vi "closed_loop_starter.vi"() -> ()   [LabVIEW 2018]
uses:
  Controls/StatisticsData.ctl
  Classes/WavefrontCorrector/WavefrontCorrector.lvclass
  Classes/CorrectionDataManager/CorrectionDataManager.lvclass
  Classes/Camera/Camera.lvclass
  Classes/WavefrontCorrectorSet/WavefrontCorrectorSet.lvclass
  Classes/Image/Image.lvclass
  Classes/ClosedLoopSmoothing/ClosedLoopSmoothing.lvclass
  Classes/HasoSlopes/HasoSlopes.lvclass
  Controls/SlopesPostProcessorList - Filter.ctl
  Controls/InteractionMatrixToCommandMatrixParameters.ctl
  Classes/Phase/Phase.lvclass
  Controls/WavefrontReconstructionMode.ctl
  Classes/Pupil/Pupil.lvclass
panel:
  in  "set_init_state_from_config_file":bool
  out "Phase values":sgl[][](graph)
  out "StatisticsData":T1
  out "Gain out":dbl min=0.0 max=1.0
  in  "Gain in":dbl min=0.0 max=1.0
  in  "Init":bool
  in  "Start Loop":bool
  in  "Exit":bool
  in  "Stop Loop":bool
  out "Camera image":u32[][](graph)
  in  "Interaction matrix file path":path
  out "error out":errorcluster
  out "ActuatorsNumber":i32
  in  "Wavefront configuration file path":path
  in  "Haso configuration file path":path
  # "This example is Hardware-dependant, \nplease use your own Haso and corrector configuration file and acquisition system, as well as your correction data backup file.\nIf you don't have a correction data backup file, please run the correction data example."
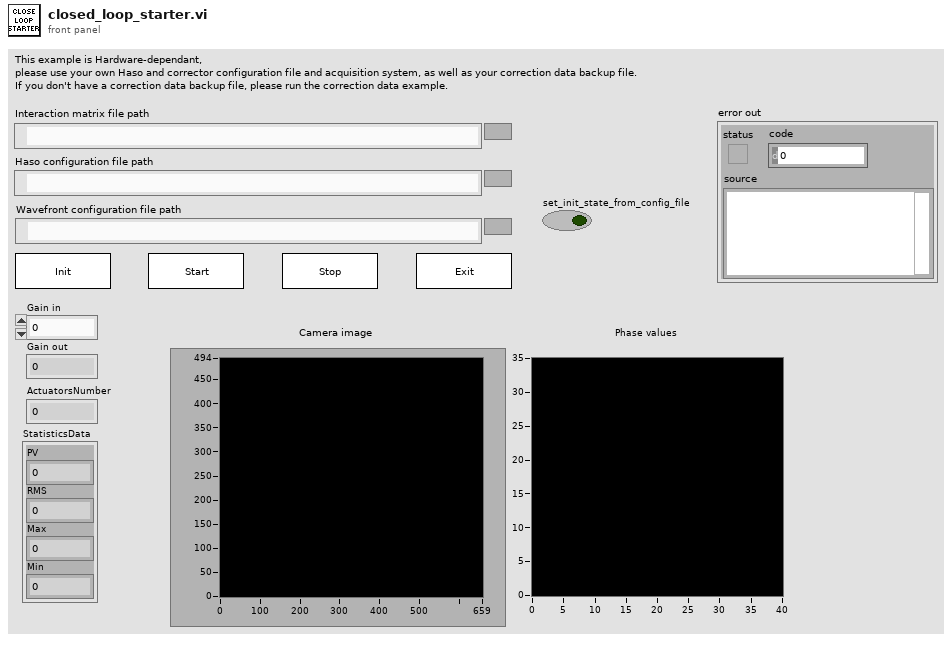
[diagram p1: front panel]
types:
  T1 = typedef "StatisticsData.ctl" = cluster{"PV":sgl, "RMS":dbl, "Max":sgl, "Min":sgl}
  T2 = typedef "SlopesPostProcessorList - Filter.ctl" = cluster{"tiltx":bool, "tilty":bool, "curv":bool, "astig0":bool, "astig45":bool, "others":bool}
  T3 = typedef "InteractionMatrixToCommandMatrixParameters.ctl" = cluster{"Number of kept modes":i32, "Tilt filtering":bool}
  T4 = typedef "WavefrontReconstructionMode.ctl" = enum16{"None", "Modal_Legendre", "Modal_Zernike", "Zonal", "Modal_Zonal_Zernike", "Modal_Zonal_Legendre"}
  T5 = typedef "HasoSpecifications.ctl" = cluster{"Serial number":string, "Revision":string, "Model":string, "Dimensions_um":T6, "Pixel position for alignment":T8, "Radius tolerance":u16, "Default start subaperture_sspp":T7, "Lower calibration wavelength_nm":dbl, "Upper calibration wavelength_nm":dbl, "Black subaperture position_sspp":T7, "TiltLimit_mrad":dbl, "Radius_m":dbl, "Smearing limit wavelength_nm":dbl, "Smearing limit exposure duration_us":dbl, "Focal_um":dbl}
  T6 = typedef "General dimensions definition.ctl" = cluster{"Size":T7, "Step":T8}
  T7 = typedef "Point2D.ctl" = cluster{"X":u32, "Y":u32}
  T8 = typedef "Point2Df.ctl" = cluster{"X":sgl, "Y":sgl}
  T9 = typedef "Data alignment enum.ctl" = enum16{"8", "16", "32"}
  T10 = typedef "Wavefront Corrector Position.ctl" = sgl[]
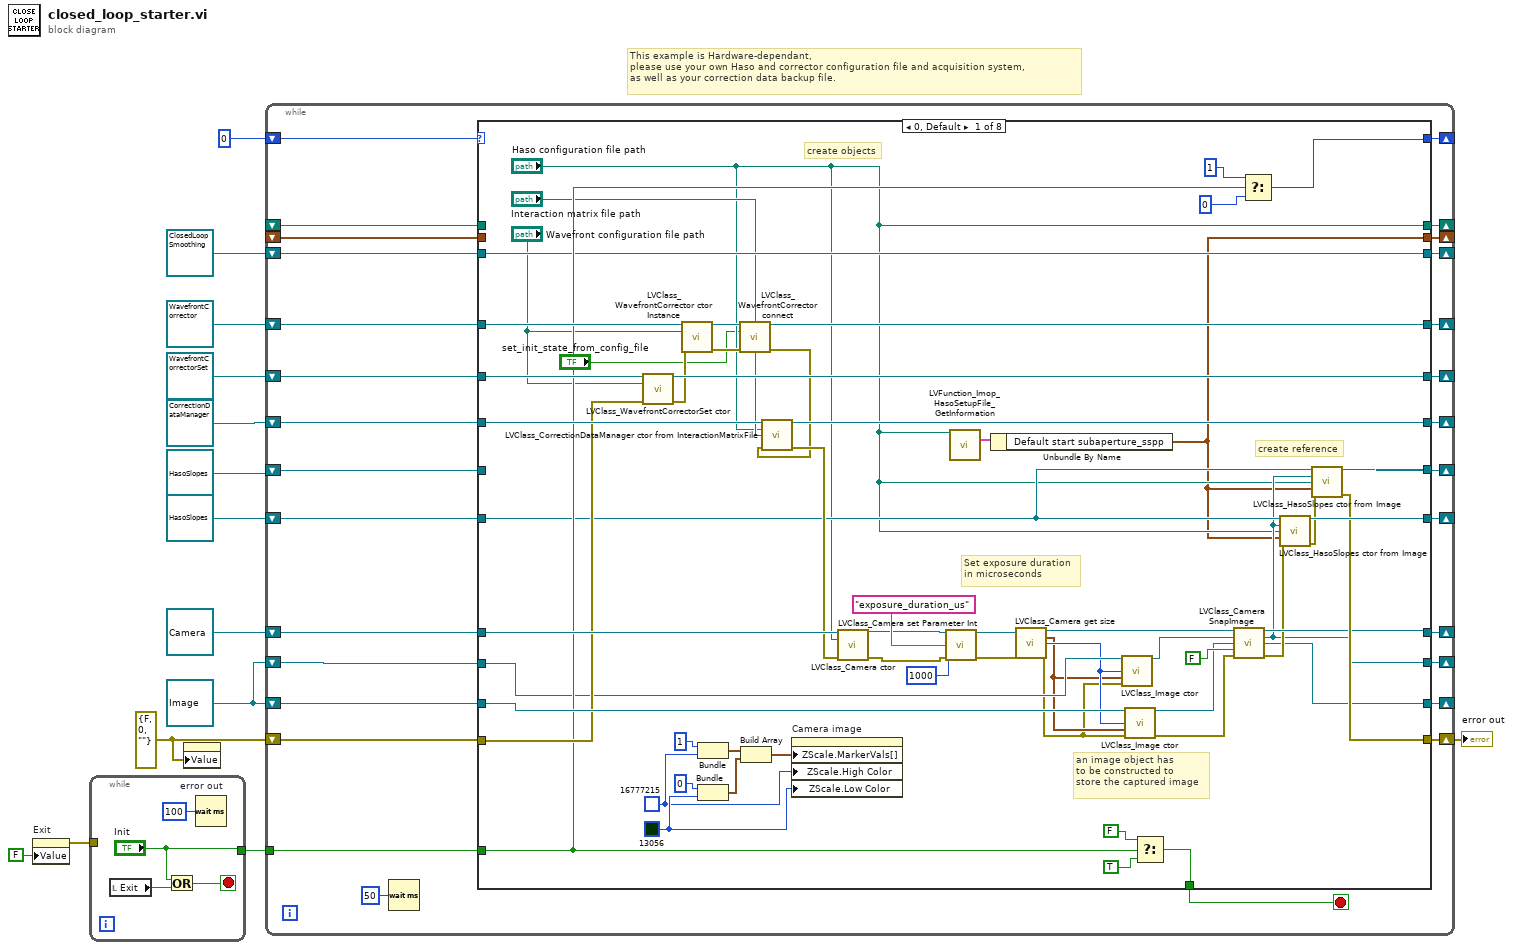
[diagram p0: block diagram]
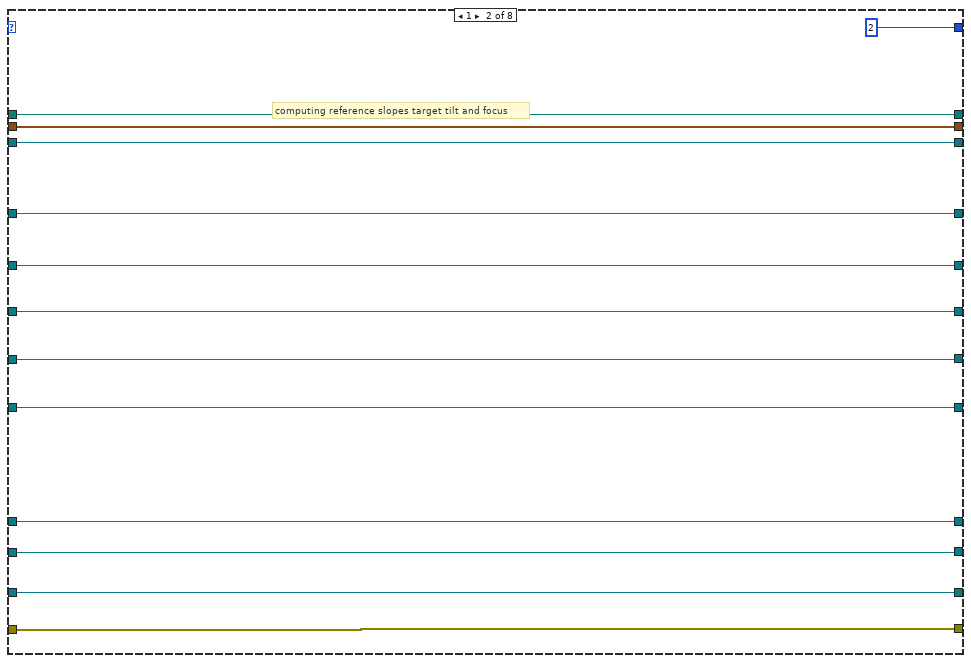
[diagram p2: hidden frame]
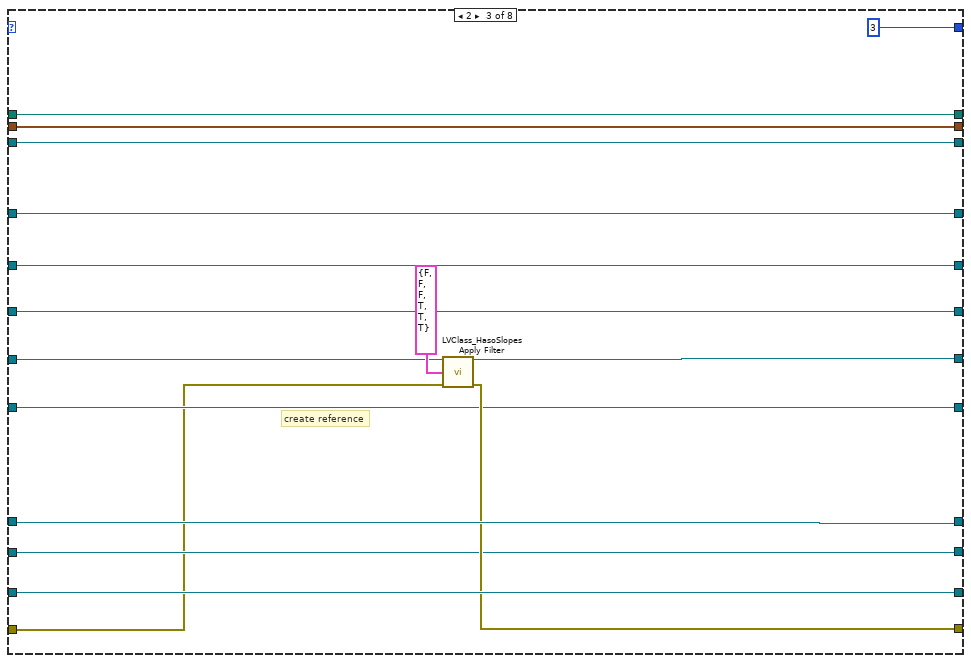
[diagram p3: hidden frame]
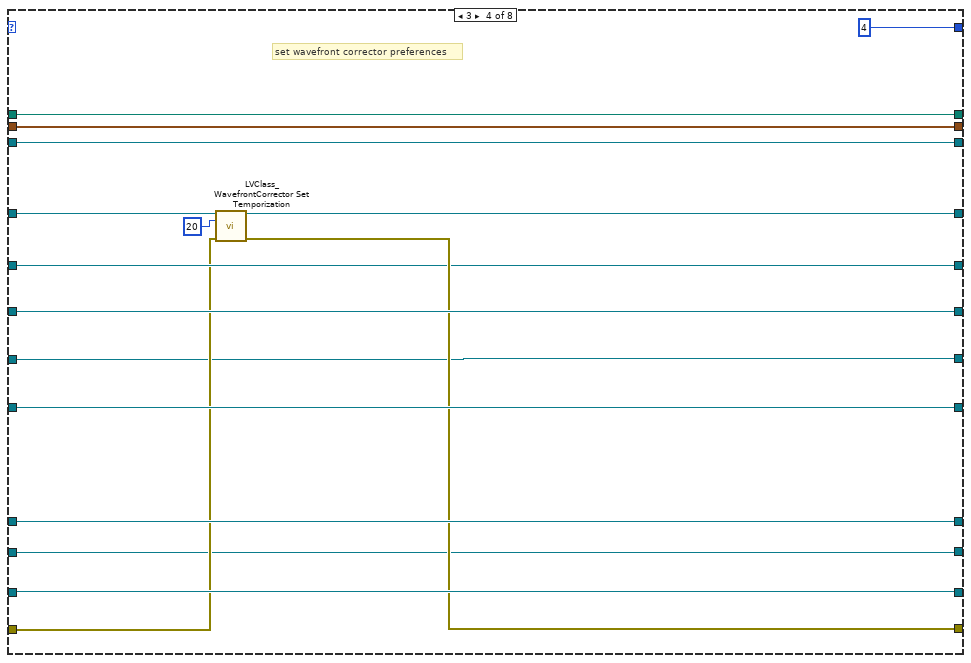
[diagram p4: hidden frame]
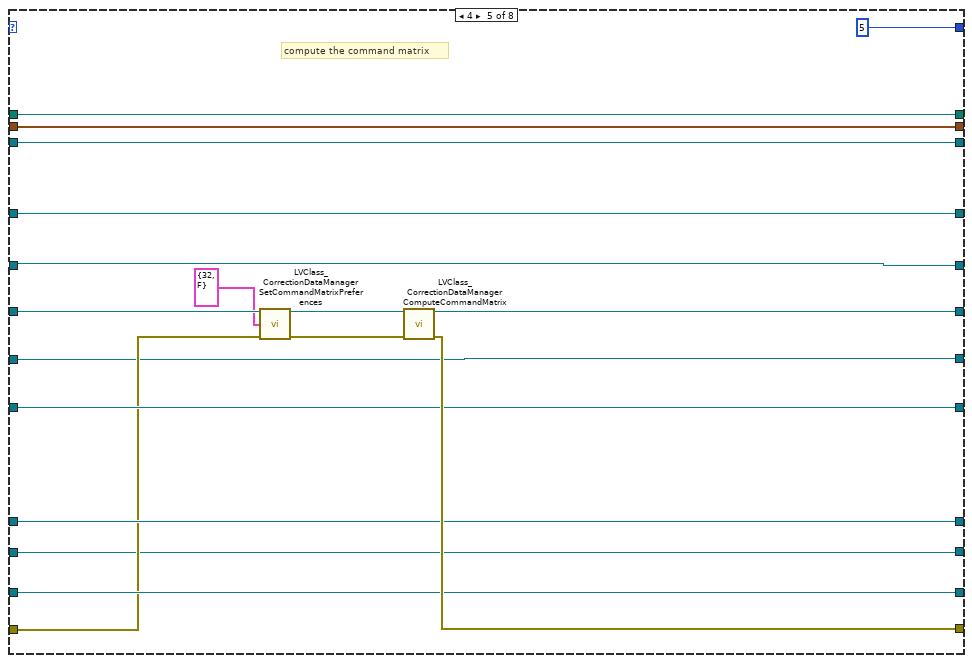
[diagram p5: hidden frame]
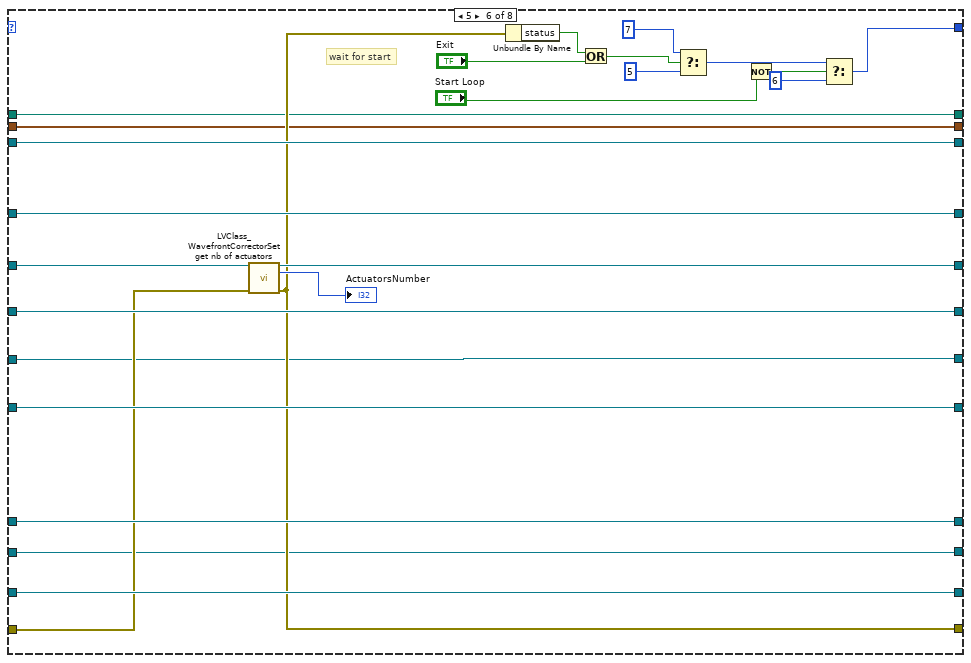
[diagram p6: hidden frame]
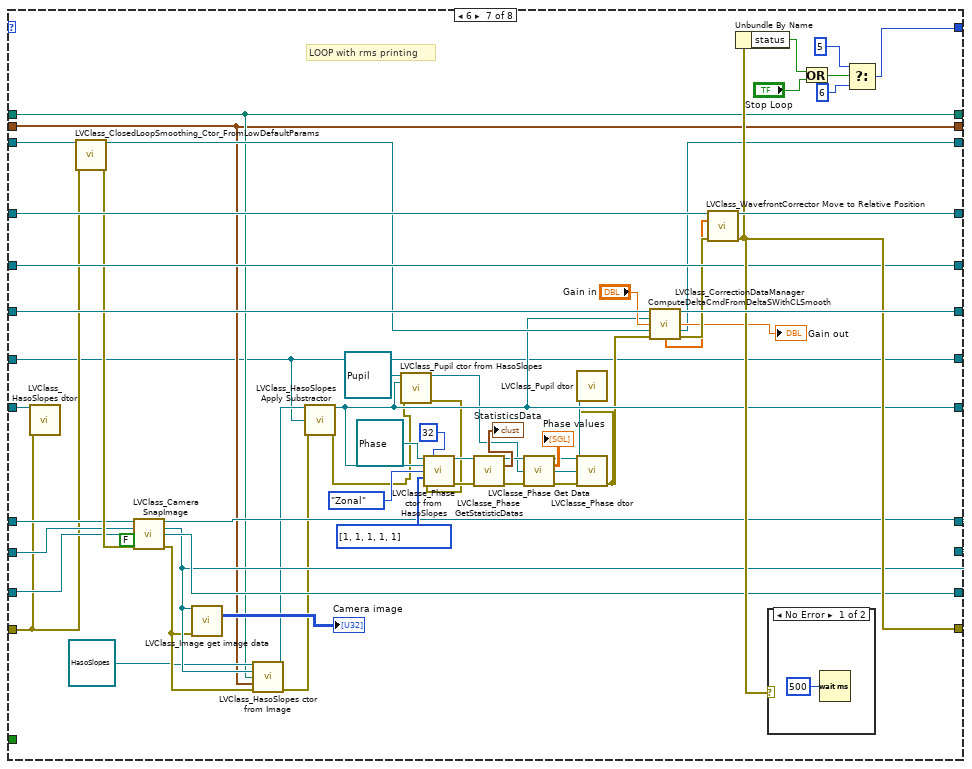
[diagram p7: hidden frame]
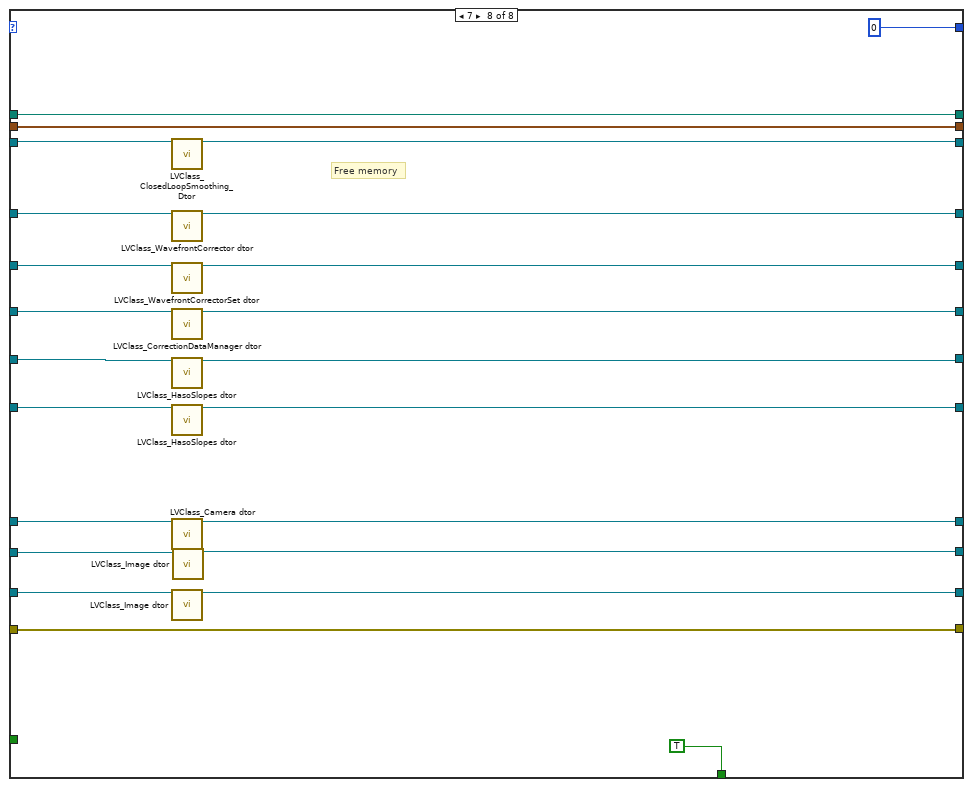
[diagram p9: hidden frame]
diagram:
  w1 = errorcluster {"status"=FALSE, "code"=0, "source"=""} ("error in (no error)")
  w3 = refnum<class "Image.lvclass"> refnum ("Image.lvclass")
  # "This example is Hardware-dependant, \nplease use your own Haso and corrector configuration file and acquisition system,\nas well as your correction data backup file."
  n1 = property on="Exit" class="Bool (strict)"("Value"=FALSE ("Exit")) -> (error out=w5:errorcluster)  [unwired: 2 in, 1 out]
  n2 = while {
    tunnel: ["Init"] -> w7
    tunnel: w5 -> [_]
    stop <- w16 stop-if-true
    n3 = local read "Exit"() -> (w17:bool)
    n4 = Or(x="Init", y=w17) -> (x .or. y?=w16:bool)
    n5 = Wait (ms)(milliseconds to wait=u32 100) -> ()  [unwired: 1 out]
  }
  n6 = property on="error out" class="Clust (strict)"("Value"=w1) -> ()  [unwired: 2 in, 2 out]
  n7 = while {
    shift-right: [w47] -> _
    shift-left: refnum<class "WavefrontCorrector.lvclass"> refnum ("WavefrontCorrector in") -> [w37]
    shift-right: [w44] -> _
    shift-left: refnum<class "CorrectionDataManager.lvclass"> refnum ("CorrectionDataManager in") -> [w36]
    shift-right: [w46] -> _
    shift-left: refnum<class "Camera.lvclass"> refnum ("Camera") -> [w43]
    shift-right: [w45] -> w9
    shift-left: w1 -> [w42]
    shift-right: [w41] -> _
    shift-left: w3 -> [w40]
    shift-right: [w39] -> _
    shift-left: refnum<class "WavefrontCorrectorSet.lvclass"> refnum ("WavefrontCorrectorSet in") -> [w38]
    shift-right: [w35] -> _
    shift-left: refnum<class "HasoSlopes.lvclass"> refnum ("HasoSlopes in") -> [w34]
    shift-right: [w32] -> _
    shift-left: 0 -> [w31]
    tunnel: w7 -> [w29]
    shift-right: [w27] -> _
    shift-left: refnum<class "ClosedLoopSmoothing.lvclass"> refnum ("ClosedLoopSmoothing.lvclass") -> [w28]
    shift-right: [w26] -> _
    shift-left: refnum<class "HasoSlopes.lvclass"> refnum ("HasoSlopes in") -> [w25]
    shift-right: [w23] -> _
    shift-left: w3 -> [w24]
    shift-right: [w22] -> _
    shift-left: _ -> [w21]
    shift-right: [w20] -> _
    shift-left: _ -> [w19]
    stop <- w33 stop-if-true
    n8 = Wait (ms)(milliseconds to wait=u32 50) -> ()  [unwired: 1 out]
    n9 = case shown="0, Default" w31 {
      tunnel: [w54 w118 w134 w150 w167 w194 w247 w268] -> w47
      tunnel: [w63 w109 w132 w146 w164 w191 w221 w264] -> w46
      tunnel: [w69 w112 w127 w145 w168 w174 w246 w260] -> w45
      tunnel: [w98 w117 w133 w149 w169 w193 w250 w267] -> w44
      tunnel: w43 -> [w103 w109 w132 w146 w164 w191 w222 w272]
      tunnel: w42 -> [w99 w112 w121 w140 w159 w175 w196 w260]
      tunnel: [w57 w111 w129 w147 w165 w190 w218 w265] -> w41
      tunnel: w40 -> [w101 w111 w129 w147 w165 w190 w217 w269]
      tunnel: [w106 w119 w135 w141 w163 w176 w245 w263] -> w39
      tunnel: w38 -> [w102 w119 w135 w141 w163 w177 w245 w270]
      tunnel: w37 -> [w100 w118 w134 w151 w167 w194 w248 w274]
      tunnel: w36 -> [w104 w117 w133 w149 w160 w193 w236 w271]
      tunnel: [w73 w116 w125 w148 w166 w192 w211 w266] -> w35
      tunnel: w34 -> [w72 w116 w125 w148 w166 w192 w202 w273]
      tunnel: [w96 _ _ _ _ _ _ TRUE] -> w33
      tunnel: [w105 2 3 4 5 w182 w249 0] -> w32
      tunnel: w29 -> [w97 _ _ _ _ _ _ _]
      tunnel: w28 -> [w95 w114 w130 w143 w157 w179 w233 w259]
      tunnel: [w95 w114 w130 w143 w157 w179 w231 w258] -> w27
      tunnel: [w71 w113 w126 w139 w155 w173 w195 w256] -> w26
      tunnel: w25 -> [_ w113 w122 w139 w155 w173 w195 w257]
      tunnel: w24 -> [w68 w110 w124 w138 w154 w172 w219 w255]
      tunnel: [w56 w110 w124 w138 w154 w172 w204 w254] -> w23
      tunnel: ["Haso configuration file path" w108 w123 w137 w153 w171 w199 w253] -> w22
      tunnel: w21 -> [_ w108 w123 w137 w153 w171 w199 w253]
      tunnel: [w49 w107 w120 w136 w152 w170 w197 w252] -> w20
      tunnel: w19 -> [_ w107 w120 w136 w152 w170 w197 w252]
      frame 0, Default {
        w88 = u32 16777215
        w92 = u32 13056
        # "create reference"
        # "Set exposure duration\nin microseconds"
        # "an image object has\nto be constructed to\nstore the captured image"
        # "create objects"
        n10 = call "LVClass_WavefrontCorrectorSet ctor.vi"("WavefrontCorrectorSet (const)"=w102, "PathToWavefrontCorrectorSetupFile"="Wavefront configuration file path", "error in (no error)"=w99) -> ("WavefrontCorrectorSet (new)"=w106:refnum<class "WavefrontCorrectorSet.lvclass">, "error out"=w87:errorcluster)  [unwired: 11 in]
        n11 = call "LVClass_WavefrontCorrector ctor Instance.vi"("WavefrontCorrector (const)"=w100, "PathToWavefrontCorrectorSetupFile"="Wavefront configuration file path", "error in (no error)"=w87) -> ("WavefrontCorrector (new)"=w55:refnum<class "WavefrontCorrector.lvclass">, "error out"=w53:errorcluster)  [unwired: 11 in]
        n12 = Bundle(1, w88) -> (w94:cluster{i32, u32})  [unwired: 1 in]
        n13 = Bundle(0, w92) -> (w93:cluster{i32, u32})  [unwired: 1 in]
        n14 = call "LVClass_WavefrontCorrector connect.vi"("WavefrontCorrector in"=w55, "set_init_state_from_config_file"="set_init_state_from_config_file", "error in (no error)"=w53) -> ("WavefrontCorrector out"=w54:refnum<class "WavefrontCorrector.lvclass">, "error out"=w52:errorcluster)  [unwired: 11 in]
        n15 = Build Array(w94, w93) -> (w91:cluster{i32, u32}[])
        n16 = call "LVClass_CorrectionDataManager ctor from InteractionMatrixFile.vi"("CorrectionDataManager (const)"=w104, "Haso config file path"="Haso configuration file path", "Interaction matrix path"="Interaction matrix file path", "error in (no error)"=w52) -> ("CorrectionDataManager (new)"=w98:refnum<class "CorrectionDataManager.lvclass">, "error out"=w84:errorcluster)  [unwired: 10 in]
        n17 = property on="Camera image" class="IntGraph (strict)"("ZScale.MarkerVals[]"=w91, "ZScale.High Color"=w88, "ZScale.Low Color"=w92) -> ()  [unwired: 2 in, 2 out]
        n18 = call "LVClass_Camera ctor.vi"("Camera (const)"=w103, "Configuration file path"="Haso configuration file path", "error in (no error)"=w84) -> ("Camera (new)"=w78:refnum<class "Camera.lvclass">, "error out"=w81:errorcluster)  [unwired: 11 in]
        n19 = call "LVClass_Camera set Parameter Int.vi"("Camera in"=w78, "parameter_name"="exposure_duration_us", "value"=1000, "error in (no error)"=w81) -> ("Camera out"=w79:refnum<class "Camera.lvclass">, "error out"=w80:errorcluster)  [unwired: 10 in]
        n20 = call "LVFunction_Imop_HasoSetupFile_GetInformation.vi"("WFS_setup_file IN"="Haso configuration file path") -> ("HASO specifications"=w51:T5)  [unwired: 10 in, 4 out]
        n21 = Unbundle By Name(w51) -> ("Default start subaperture_sspp"=w49:T7)
        n22 = call "LVClass_Camera get size.vi"("Camera in"=w79, "error in (no error)"=w80) -> ("Camera out"=w64:refnum<class "Camera.lvclass">, "size"=w66:T7, "Number of bits"=w67:T9, "error out"=w65:errorcluster)  [unwired: 10 in]
        n23 = call "LVClass_Image ctor.vi"("Image (const)"=w68, "Data alignment"=w67, "Size"=w66, "error in (no error)"=w65) -> ("Image (new)"=w62:refnum<class "Image.lvclass">)  [unwired: 10 in, 1 out]
        n24 = call "LVClass_Image ctor.vi"("Image (const)"=w101, "Data alignment"=w67, "Size"=w66, "error in (no error)"=w65) -> ("Image (new)"=w58:refnum<class "Image.lvclass">, "error out"=w60:errorcluster)  [unwired: 10 in]
        n25 = Select(t=FALSE, s=w97, f=TRUE) -> (s? t:f=w96:bool)
        n26 = call "LVClass_Camera SnapImage.vi"("Camera in"=w64, "Image"=w62, "Image RAW"=w58, "remove_background"=FALSE, "error in (no error)"=w60) -> ("Camera out"=w63:refnum<class "Camera.lvclass">, "Image (dup)"=w56:refnum<class "Image.lvclass">, "Image (dup) RAW"=w57:refnum<class "Image.lvclass">, "error out"=w59:errorcluster)  [unwired: 7 in]
        n27 = Select(t=1, s=w97, f=0) -> (s? t:f=w105:i32)
        n28 = call "LVClass_HasoSlopes ctor from Image.vi"("HasoSlopes (const)"=w72, "Image"=w56, "Haso configuration file"="Haso configuration file path", "start subpupil"=w49, "error in (no error)"=w59) -> ("HasoSlopes (new)"=w73:refnum<class "HasoSlopes.lvclass">, "error out"=w70:errorcluster)  [unwired: 8 in, 1 out]
        n29 = call "LVClass_HasoSlopes ctor from Image.vi"("HasoSlopes (const)"=w72, "Image"=w56, "Haso configuration file"="Haso configuration file path", "start subpupil"=w49, "error in (no error)"=w70) -> ("HasoSlopes (new)"=w71:refnum<class "HasoSlopes.lvclass">, "error out"=w69:errorcluster)  [unwired: 8 in, 1 out]
      }
      frame 1 {
        # "computing reference slopes target tilt and focus"
      }
      frame 2 {
        # "create reference"
        n30 = call "LVClass_HasoSlopes Apply Filter.vi"("HasoSlopes in"=w122, "filter"=T2 {"tiltx"=FALSE, "tilty"=FALSE, "curv"=FALSE, "astig0"=TRUE, "astig45"=TRUE, "others"=TRUE} ("Filter"), "error in (no error)"=w121) -> ("HasoSlopes out"=w126:refnum<class "HasoSlopes.lvclass">, "error out"=w127:errorcluster)  [unwired: 11 in]
      }
      frame 3 {
        # "set wavefront corrector preferences"
        n31 = call "LVClass_WavefrontCorrector Set Temporization.vi"("WavefrontCorrector in"=w151, "Sleep after command apply (ms)"=20 ("Sleep after command apply_ms"), "error in (no error)"=w140) -> ("WavefrontCorrector out"=w150:refnum<class "WavefrontCorrector.lvclass">, "error out"=w145:errorcluster)  [unwired: 11 in]
      }
      frame 4 {
        # "compute the command matrix"
        n32 = call "LVClass_CorrectionDataManager SetCommandMatrixPreferences.vi"("CorrectionDataManager in"=w160, "Prefs"=T3 {"Number of kept modes"=32, "Tilt filtering"=FALSE}, "error in (no error)"=w159) -> ("CorrectionDataManager out"=w161:refnum<class "CorrectionDataManager.lvclass">, "error out"=w158:errorcluster)  [unwired: 11 in]
        n33 = call "LVClass_CorrectionDataManager ComputeCommandMatrix.vi"("CorrectionDataManager in"=w161, "error in (no error)"=w158) -> ("CorrectionDataManager out"=w169:refnum<class "CorrectionDataManager.lvclass">, "error out"=w168:errorcluster)  [unwired: 12 in]
      }
      frame 5 {
        # "wait for start"
        n34 = call "LVClass_WavefrontCorrectorSet get nb of actuators.vi"("WavefrontCorrectorSet in"=w177, "error in (no error)"=w175) -> ("WavefrontCorrectorSet out"=w176:refnum<class "WavefrontCorrectorSet.lvclass">, "ActuatorsNumber"=→"ActuatorsNumber":i32, "error out"=w174:errorcluster)  [unwired: 11 in]
        n35 = Unbundle By Name(w174) -> ("status"=w184:bool)
        n36 = Or(x=w184, y="Exit") -> (x .or. y?=w187:bool)
        n37 = Select(t=7, s=w187, f=5) -> (s? t:f=w183:i32)
        n38 = Not(x="Start Loop") -> (.not. x?=w180:bool)
        n39 = Select(t=w183, s=w180, f=6) -> (s? t:f=w182:i32)
      }
      frame 6 {
        # "LOOP with rms printing"
        n40 = call "LVClass_HasoSlopes dtor.vi"("HasoSlopes in"=w202, "error in (no error)"=w196) -> ()  [unwired: 12 in, 2 out]
        n41 = call "LVClass_ClosedLoopSmoothing_Ctor_FromLowDefaultParams.vi"("ClosedLoopSmoothing in"=w233, "error in (no error)"=w196) -> ("ClosedLoopSmoothing out"=w232:refnum<class "ClosedLoopSmoothing.lvclass">, "error out"=w223:errorcluster)  [unwired: 12 in]
        n42 = call "LVClass_Camera SnapImage.vi"("Camera in"=w222, "Image"=w219, "Image RAW"=w217, "remove_background"=FALSE, "error in (no error)"=w223) -> ("Camera out"=w221:refnum<class "Camera.lvclass">, "Image (dup)"=w204:refnum<class "Image.lvclass">, "Image (dup) RAW"=w218:refnum<class "Image.lvclass">, "error out"=w203:errorcluster)  [unwired: 7 in]
        n43 = call "LVClass_Image get image data.vi"("Image in"=w204, "error in (no error)"=w203) -> ("Image data out"=→"Camera image":u32[][])  [unwired: 11 in, 2 out]
        n44 = call "LVClass_HasoSlopes ctor from Image.vi"("HasoSlopes (const)"=refnum<class "HasoSlopes.lvclass"> refnum ("HasoSlopes in"), "Image"=w204, "Haso configuration file"=w199, "start subpupil"=w197, "error in (no error)"=w203) -> ("HasoSlopes (new)"=w198:refnum<class "HasoSlopes.lvclass">, "error out"=w201:errorcluster)  [unwired: 8 in, 1 out]
        n45 = call "LVClass_HasoSlopes Apply Substractor.vi"("HasoSlopes in"=w198, "HasoSlopes to substract"=w195, "error in (no error)"=w201) -> ("HasoSlopes out"=w211:refnum<class "HasoSlopes.lvclass">, "error out"=w208:errorcluster)  [unwired: 11 in]
        n46 = call "LVClass_Pupil ctor from HasoSlopes.vi"("Pupil (const)"=refnum<class "Pupil.lvclass"> refnum ("Pupil in"), "HasoSlopes"=w211, "error in (no error)"=w208) -> ("Pupil (new)"=w210:refnum<class "Pupil.lvclass">, "error out"=w207:errorcluster)  [unwired: 10 in, 1 out]
        n47 = call "LVClasse_Phase ctor from HasoSlopes.vi"("Phase (const)"=refnum<class "Phase.lvclass"> refnum ("Phase in"), "Number of coefficients"=u8 32, "HasoSlopes"=w211, "TypePhase"=WavefrontReconstructionMode."Zonal", "Filter"=u8[] [1, 1, 1, 1, 1], "error in (no error)"=w207) -> ("Phase (new)"=w226:refnum<class "Phase.lvclass">, "error out"=w225:errorcluster)  [unwired: 7 in, 1 out]
        n48 = call "LVClasse_Phase GetStatisticDatas.vi"("Phase in"=w226, "error in (no error)"=w225) -> ("Phase out"=w215:refnum<class "Phase.lvclass">, "StatisticsData"=→"StatisticsData":T1, "error out"=w213:errorcluster)  [unwired: 11 in]
        n49 = call "LVClasse_Phase Get Data.vi"("Phase in"=w215, "Pupil"=w210, "error in (no error)"=w213) -> ("Phase out"=w214:refnum<class "Phase.lvclass">, "data"=→"Phase values":sgl[][], "Pupil (dup)"=w209:refnum<class "Pupil.lvclass">, "error out"=w206:errorcluster)  [unwired: 9 in]
        n50 = call "LVClasse_Phase dtor.vi"("Phase in"=w214, "error in (no error)"=w206) -> ("error out"=w205:errorcluster)  [unwired: 12 in, 1 out]
        n51 = call "LVClass_Pupil dtor.vi"("Pupil in"=w209, "error in (no error)"=w205) -> ()  [unwired: 12 in, 2 out]
        n52 = call "LVClass_CorrectionDataManager ComputeDeltaCmdFromDeltaSWithCLSmooth.vi"("CorrectionDataManager in"=w236, "Delta Slopes IN"=w211, "Gain in"="Gain in", "ClosedLoopSmoothing in"=w232, "error in (no error)"=w205) -> ("CorrectionDataManager out"=w250:refnum<class "CorrectionDataManager.lvclass">, "Gain out"=→"Gain out":dbl, "ClosedLoopSmoothing out"=w231:refnum<class "ClosedLoopSmoothing.lvclass">, "DeltaPosition"=w241:T10, "error out"=w242:errorcluster)  [unwired: 5 in, 1 out]
        n53 = call "LVClass_WavefrontCorrector Move to Relative Position.vi"("WavefrontCorrector in"=w248, "Wavefront Relative Position"=w241, "error in (no error)"=w242) -> ("WavefrontCorrector out"=w247:refnum<class "WavefrontCorrector.lvclass">, "error out"=w246:errorcluster)  [unwired: 11 in]
        n54 = Unbundle By Name(w246) -> ("status"=w239:bool)
        n55 = case shown="No Error" w246 {
          frame No Error {
            n56 = Wait (ms)(milliseconds to wait=u32 500) -> ()  [unwired: 1 out]
          }
          frame Error {
          }
        }
        n57 = Or(x=w239, y="Stop Loop") -> (x .or. y?=w238:bool)
        n58 = Select(t=5, s=w238, f=6) -> (s? t:f=w249:i32)
      }
      frame 7 {
        # "Free memory"
        n59 = call "LVClass_ClosedLoopSmoothing_Dtor.vi"("ClosedLoopSmoothing in"=w259) -> ("ClosedLoopSmoothing out"=w258:refnum<class "ClosedLoopSmoothing.lvclass">)  [unwired: 13 in, 1 out]
        n60 = call "LVClass_WavefrontCorrector dtor.vi"("WavefrontCorrector in"=w274) -> ("WavefrontCorrector out"=w268:refnum<class "WavefrontCorrector.lvclass">)  [unwired: 13 in, 1 out]
        n61 = call "LVClass_WavefrontCorrectorSet dtor.vi"("WavefrontCorrectorSet in"=w270) -> ("WavefrontCorrectorSet out"=w263:refnum<class "WavefrontCorrectorSet.lvclass">)  [unwired: 13 in, 1 out]
        n62 = call "LVClass_CorrectionDataManager dtor.vi"("CorrectionDataManager in"=w271) -> ("CorrectionDataManager out"=w267:refnum<class "CorrectionDataManager.lvclass">)  [unwired: 13 in, 1 out]
        n63 = call "LVClass_HasoSlopes dtor.vi"("HasoSlopes in"=w257) -> ("HasoSlopes out"=w256:refnum<class "HasoSlopes.lvclass">)  [unwired: 13 in, 1 out]
        n64 = call "LVClass_HasoSlopes dtor.vi"("HasoSlopes in"=w273) -> ("HasoSlopes out"=w266:refnum<class "HasoSlopes.lvclass">)  [unwired: 13 in, 1 out]
        n65 = call "LVClass_Camera dtor.vi"("Camera in"=w272) -> ("Camera out"=w264:refnum<class "Camera.lvclass">)  [unwired: 13 in, 1 out]
        n66 = call "LVClass_Image dtor.vi"("Image in"=w269) -> ("Image out"=w265:refnum<class "Image.lvclass">)  [unwired: 13 in, 1 out]
        n67 = call "LVClass_Image dtor.vi"("Image in"=w255) -> ("Image out"=w254:refnum<class "Image.lvclass">)  [unwired: 13 in, 1 out]
      }
    }
  }
  "error out" <- w9
